vi "enableDisableSLMbuttons.vi"(9 "Active":u16, 11 "Radio":u16) -> (0 "Semi":T1(ring), 1 "ModType":T1(ring), 2 "Phase":T1(ring), 3 "Trans":T1(ring), 4 "HoloCode":T1(ring), 5 "PrefabrHolo":T1(ring), 6 "just ON/OFF":T1(ring))   [LabVIEW 2023]
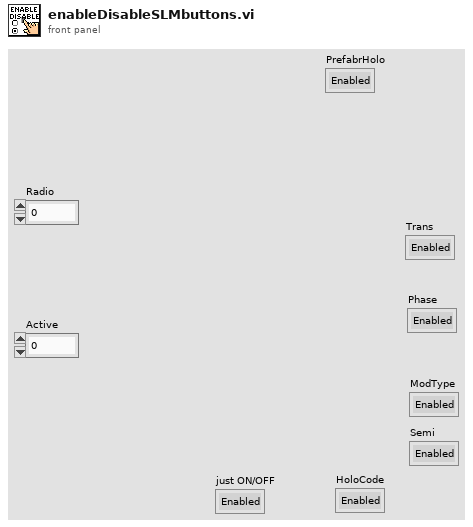
[diagram p1: front panel]
types:
  T1 = enum8{"Enabled", "Disabled", "Disabled and Grayed Out"}
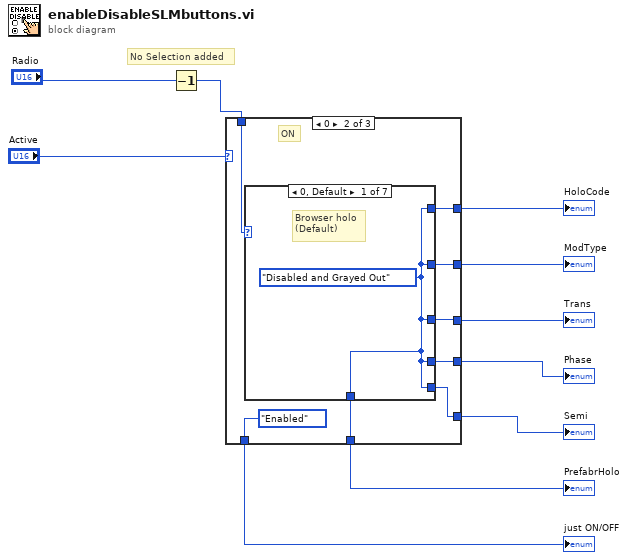
[diagram p0: block diagram]
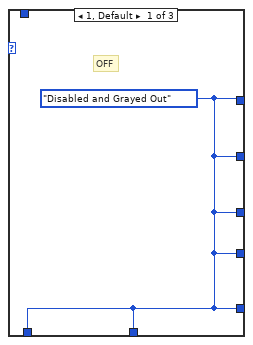
[diagram p2: hidden frame]
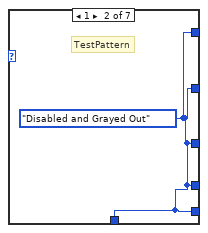
[diagram p3: hidden frame]
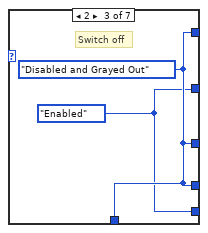
[diagram p4: hidden frame]
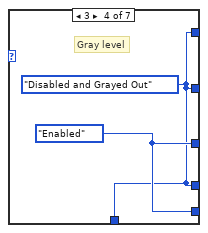
[diagram p5: hidden frame]
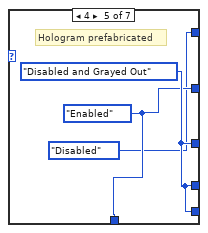
[diagram p6: hidden frame]
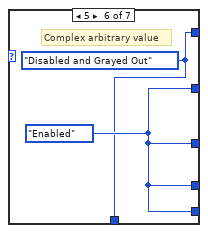
[diagram p7: hidden frame]
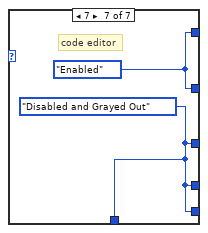
[diagram p8: hidden frame]
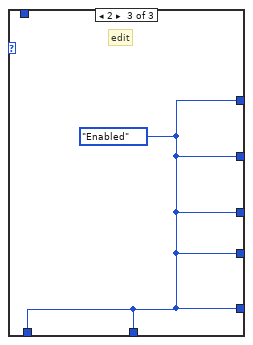
[diagram p9: hidden frame]
diagram:
  # "No Selection added"
  n1 = Decrement(x="Radio") -> (x-1=w2:u16)
  n2 = case shown="0" "Active" {
    tunnel: [w11 w19 w33] -> w5
    tunnel: [w11 w18 w33] -> w6
    tunnel: [w11 w13 w33] -> w8
    tunnel: [w11 w17 w33] -> w9
    tunnel: [w11 w16 w33] -> w7
    tunnel: [w11 w15 w33] -> w10
    tunnel: [w11 T1."Enabled" ("Disabled") w33] -> w3
    tunnel: w2 -> [_ w12 _]
    frame 1, Default {
      w11 = T1."Disabled and Grayed Out" ("Disabled")
      # "OFF"
    }
    frame 0 {
      # "ON"
      n3 = case shown="0, Default" w12 {
        tunnel: [w20 w21 w23 w24 T1."Disabled" ("Disabled") w29 w32] -> w19
        tunnel: [w20 w21 w22 w24 w27 w30 w32] -> w18
        tunnel: [w20 w21 w23 w25 w28 w30 w31] -> w13
        tunnel: [w20 w21 w23 w24 w28 w30 w31] -> w17
        tunnel: [w20 w21 w22 w25 w28 w30 w31] -> w16
        tunnel: [w20 w21 w23 w24 w27 w29 w31] -> w15
        frame 0, Default {
          w20 = T1."Disabled and Grayed Out" ("Disabled")
          # "Browser holo\n(Default)"
        }
        frame 1 {
          w21 = T1."Disabled and Grayed Out" ("Disabled")
          # "TestPattern"
        }
        frame 2 {
          w23 = T1."Disabled and Grayed Out" ("Disabled")
          w22 = T1."Enabled" ("Disabled")
          # "Switch off"
        }
        frame 3 {
          w25 = T1."Enabled" ("Disabled")
          w24 = T1."Disabled and Grayed Out" ("Disabled")
          # "Gray level"
        }
        frame 4 {
          w27 = T1."Enabled" ("Disabled")
          w28 = T1."Disabled and Grayed Out" ("Disabled")
          # "Hologram prefabricated"
        }
        frame 5 {
          w29 = T1."Disabled and Grayed Out" ("Disabled")
          w30 = T1."Enabled" ("Disabled")
          # "Complex arbitrary value"
        }
        frame 7 {
          w31 = T1."Disabled and Grayed Out" ("Disabled")
          w32 = T1."Enabled" ("Disabled")
          # "code editor"
        }
      }
    }
    frame 2 {
      w33 = T1."Enabled" ("Disabled")
      # "edit"
    }
  }
  "PrefabrHolo" <- w10
  "Phase" <- w9
  "Trans" <- w8
  "Semi" <- w7
  "ModType" <- w6
  "HoloCode" <- w5
  "just ON/OFF" <- w3
